vi "convertBB_FW.vi"(8 "Numeric [3]":u32, 9 "Numeric [2]":u32, 10 "Numeric [1]":u32, 11 "Numeric [0]":u32) -> (3 "BB FW":string)   [LabVIEW 2018]
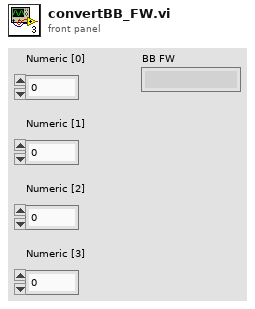
[diagram p1: front panel]
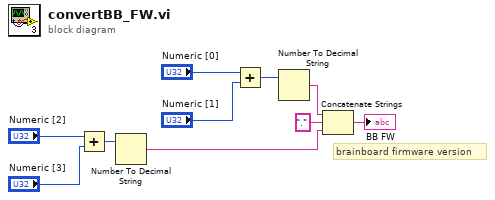
[diagram p0: block diagram]
diagram:
  # "brainboard firmware version"
  n1 = Add(x="Numeric [2]", y="Numeric [3]") -> (x+y=w2:u32)
  n2 = Number To Decimal String(number=w2) -> (decimal integer string=w4:string)  [unwired: 1 in]
  n3 = Add(x="Numeric [0]", y="Numeric [1]") -> (x+y=w1:u32)
  n4 = Number To Decimal String(number=w1) -> (decimal integer string=w3:string)  [unwired: 1 in]
  n5 = Concatenate Strings(w3, "." ("string"), w4) -> (→"BB FW":string)
